vi "LED-Set Text_Label.vi"() -> (4 "\"Set Text\" Label":string)   [LabVIEW 2012, in "LED Display.xctl"]
doc: "This VI will set the string value to \"Set Text\". It replaced teh constant to avoid easy modification of the string value and facilitating the translation to another language."
uses:
  LED Display.xctl
panel:
  in  "String":string="Set Text"
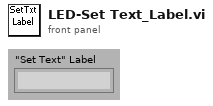
[diagram p1: front panel]
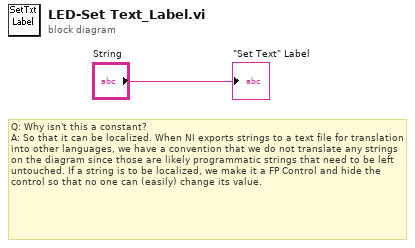
[diagram p0: block diagram]
diagram:
  # "Q: Why isn't this a constant?\nA: So that it can be localized. When NI exports strings to a text file for translation into other languages, we have a convention that we do not translate any strings on the diagram since those are likely programmatic strings that need to be left untouched. If a string is to be localized, we make it a FP Control and hide the control so that no one can (easily) change its value."
  "\"Set Text\" Label" <- "String"
